vi "GetParam.vi"(8 "error in (no error)":errorcluster caption="entrée d'erreur (pas d'erreur)", 11 "label_binarize.lvclass":refnum<class "label_binarize.lvclass">) -> (0 "error out":errorcluster caption="sortie d'erreur", 2 "label_binarize":T1={"classes"=[], "neg_label"=0, "pos_label"=1, "sparse_output"=FALSE}, 3 "label_binarize.lvclass":refnum<class "label_binarize.lvclass">)   [LabVIEW 2020, in "label_binarize.lvclass"]
doc: "Get Parameters"
uses:
  label_binarize.lvclass
  label_binarize.lvclass/label_binarize.ctl
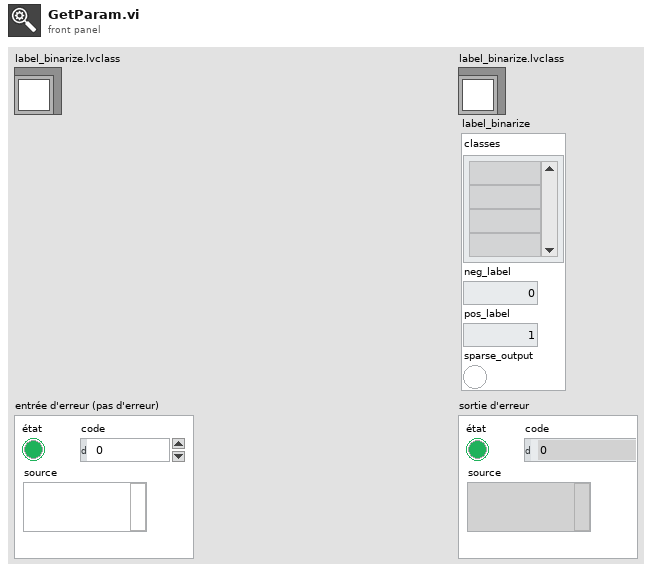
[diagram p1: front panel]
types:
  T1 = cluster{"classes":string[][], "neg_label":i32, "pos_label":i32, "sparse_output":bool}
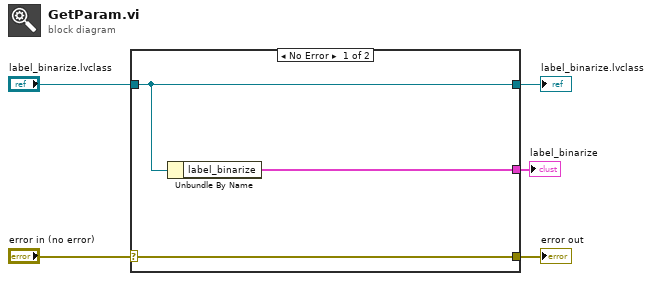
[diagram p0: block diagram]
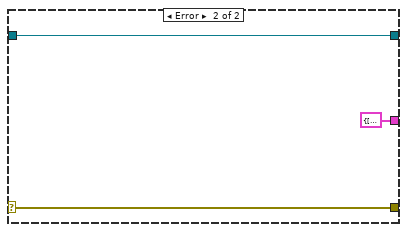
[diagram p2: hidden frame]
diagram:
  n1 = case shown="No Error" "error in (no error)" {
    selector: "error in (no error)" -> [w8 w10]
    tunnel: [w8 w10] -> w4
    tunnel: [w7 w11] -> w2
    tunnel: "label_binarize.lvclass" -> [w7 w11]
    tunnel: [w6 T1 {"classes"=[], "neg_label"=0, "pos_label"=0, "sparse_output"=FALSE} ("label_binarize")] -> w1
    frame No Error {
      n2 = Unbundle By Name(w7) -> ("label_binarize"=w6:T1)
    }
    frame Error {
    }
  }
  "error out" <- w4
  "label_binarize.lvclass" <- w2
  "label_binarize" <- w1
